vi "Autosize Listbox Columns (Uniform Text).vi"(4 "error in (no error)":errorcluster, 6 "Resize Table?":bool, 7 "Table Ref":refnum<vi>) -> (0 "error out":errorcluster, 3 "Table Ref (dup)":refnum<vi>)   [LabVIEW 2017, in "UI-DisplayTable(dev).xctl"]
doc: "This VI resizes each column of the table specified by Table Ref based on the widest entry of the column. Additionally, if Resize Table? is TRUE, the VI will set the table width based on the number of populated columns."
uses:
  UI-DisplayTable(dev).xctl
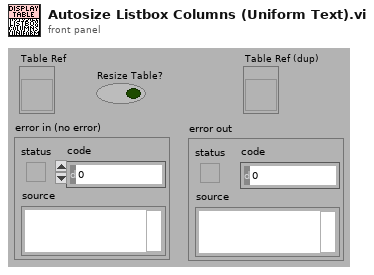
[diagram p1: front panel]
types:
  T1 = enum16{"User-specified Font", "Application Font", "System Font", "Dialog Font"}
  T2 = cluster{"Font Name:":string, "Size":i16, "Strikeout?":bool, "Italic?":bool, "Underline?":bool, "Outline?":bool, "Shadow?":bool, "Bold?":bool}
  T3 = cluster{"left":i16, "top":i16, "right":i16, "bottom":i16}
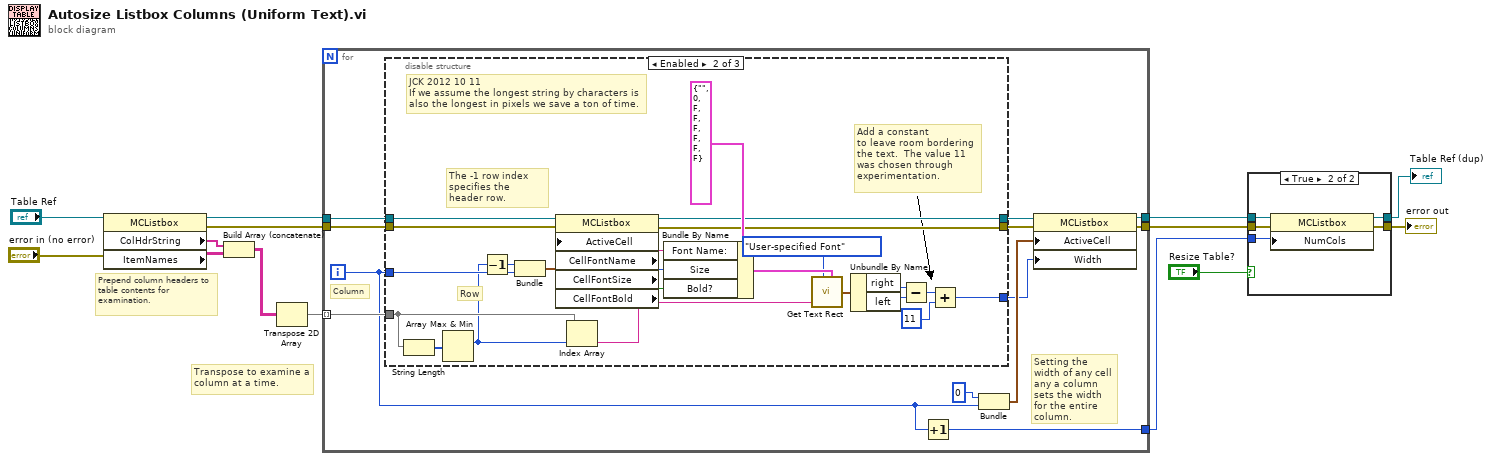
[diagram p0: block diagram]
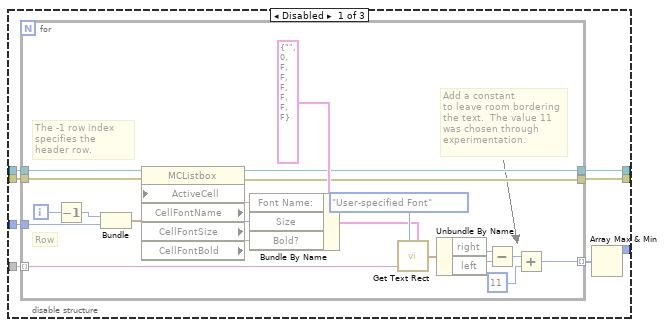
[diagram p3: hidden frame]
diagram:
  # "Transpose to examine a column at a time."
  # "Prepend column headers to table contents for examination."
  n1 = property class="MCListbox"(reference="Table Ref", error in="error in (no error)") -> (reference out=w14:refnum<vi>, error out=w10:errorcluster, "ColHdrString"=w13:string[], "ItemNames"=w9:string[][])
  n2 = Build Array (concatenate)(w13, w9) -> (w12:string[][])
  n3 = Transpose 2D Array(2D array=w12) -> (transposed array=w11:string[][])
  n4 = for {
    tunnel: w11 -> [w26] mode=indexing
    tunnel: w14 -> [w25]
    tunnel: w10 -> [w24]
    tunnel: [w18] -> w4
    tunnel: [w17] -> w5
    tunnel: [w15] -> w3
    i -> [w16]
    # "Setting the width of any cell any a column sets the width for the entire column."
    # "Column"
    n5 = disable-structure shown="Enabled" {
      disable-tunnel: w26 -> [w34 w63 _]
      disable-tunnel: w25 -> [w33 w60 _]
      disable-tunnel: w24 -> [w31 w59 _]
      disable-tunnel: [w30 w58 _] -> w23
      disable-tunnel: [w29 w57 _] -> w22
      disable-tunnel: [w28 w56 _] -> w19
      disable-tunnel: w16 -> [w27 w64 _]
      frame Disabled {
        n6 = for {
          tunnel: w34 -> [w47] mode=indexing
          tunnel: w33 -> [w55]
          tunnel: w27 -> [w54]
          tunnel: [w36] -> w32 mode=indexing
          tunnel: w31 -> [w41]
          tunnel: [w40] -> w29
          tunnel: [w39] -> w30
          i -> [w43]
          # "The -1 row index specifies the header row."
          # "Add a constant\nto leave room bordering the text.  The value 11 was chosen through experimentation."
          # "Row"
          n7 = Decrement(x=w43) -> (x-1=w42:i32)
          n8 = Bundle(w42, w54) -> (w53:cluster{i32, i32})  [unwired: 1 in]
          n9 = property class="MCListbox"(reference=w55, error in=w41, "ActiveCell"=w53) -> (reference out=w39:refnum<vi>, error out=w40:errorcluster, "CellFontName"=w51:string, "CellFontSize"=w37:u32, "CellFontBold"=w50:bool)
          n10 = Bundle By Name(cluster=T2 {"Font Name:"="", "Size"=0, "Strikeout?"=FALSE, "Italic?"=FALSE, "Underline?"=FALSE, "Outline?"=FALSE, "Shadow?"=FALSE, "Bold?"=FALSE} ("[user-specified font]"), "Font Name:"=w51, "Size"=w37, "Bold?"=w50) -> (w48:T2)
          n11 = call <vilib>:"Get Text Rect.vi"("desired font(Application)"=T1."User-specified Font", "text"=w47, "[user-specified font]"=w48) -> ("rect"=w46:T3)  [unwired: 6 in]
          n12 = Unbundle By Name(w46) -> ("right"=w45:i16, "left"=w44:i16)
          n13 = Subtract(x=w45, y=w44) -> (x-y=w38:i16)
          n14 = Add(x=w38, y=i16 11) -> (x+y=w36:i16)
        }
        n15 = Array Max & Min(array=w32) -> (max value=w28:i16)  [unwired: 3 out]
      }
      frame Enabled {
        # "JCK 2012 10 11\nIf we assume the longest string by characters is also the longest in pixels we save a ton of time."
        # "The -1 row index specifies the header row."
        # "Add a constant\nto leave room bordering the text.  The value 11 was chosen through experimentation."
        # "Row"
        n16 = String Length(string=w63) -> (length=w78:i32[])
        n17 = Array Max & Min(array=w78) -> (max index (indices)=w62:i32)  [unwired: 3 out]
        n18 = Decrement(x=w62) -> (x-1=w74:i32)
        n19 = Bundle(w74, w64) -> (w65:cluster{i32, i32})  [unwired: 1 in]
        n20 = property class="MCListbox"(reference=w60, error in=w59, "ActiveCell"=w65) -> (reference out=w58:refnum<vi>, error out=w57:errorcluster, "CellFontName"=w67:string, "CellFontSize"=w76:u32, "CellFontBold"=w68:bool)
        n21 = Index Array(array=w63, index=w62) -> (element=w61:string)
        n22 = Bundle By Name(cluster=T2 {"Font Name:"="", "Size"=0, "Strikeout?"=FALSE, "Italic?"=FALSE, "Underline?"=FALSE, "Outline?"=FALSE, "Shadow?"=FALSE, "Bold?"=FALSE} ("[user-specified font]"), "Font Name:"=w67, "Size"=w76, "Bold?"=w68) -> (w70:T2)
        n23 = call <vilib>:"Get Text Rect.vi"("desired font(Application)"=T1."User-specified Font", "text"=w61, "[user-specified font]"=w70) -> ("rect"=w71:T3)  [unwired: 6 in]
        n24 = Unbundle By Name(w71) -> ("right"=w72:i16, "left"=w73:i16)
        n25 = Subtract(x=w72, y=w73) -> (x-y=w75:i16)
        n26 = Add(x=w75, y=i16 11) -> (x+y=w56:i16)
      }
      frame Disabled {
      }
    }
    n27 = Increment(x=w16) -> (x+1=w15:i32)
    n28 = Bundle(0, w16) -> (w20:cluster{i32, i32})  [unwired: 1 in]
    n29 = property class="MCListbox"(reference=w23, error in=w22, "ActiveCell"=w20, "Width"=w19) -> (reference out=w17:refnum<vi>, error out=w18:errorcluster)
  }
  n30 = case shown="True" "Resize Table?" {
    tunnel: w5 -> [w79 w85]
    tunnel: w4 -> [w80 w84]
    tunnel: w3 -> [_ w83]
    tunnel: [w80 w82] -> w2
    tunnel: [w79 w81] -> w1
    frame False {
    }
    frame True {
      n31 = property class="MCListbox"(reference=w85, error in=w84, "NumCols"=w83) -> (reference out=w81:refnum<vi>, error out=w82:errorcluster)
    }
  }
  "error out" <- w2
  "Table Ref (dup)" <- w1
